vi "Lab Panel V5.24.2.vi"() -> ()   [LabVIEW 2013] (continued)
            n3236 = global read "Global display 3.vi" "log 1-1"() -> (→"LOG LAB01-1":string)
            n3237 = global read "Global display 3.vi" "log 3-1"() -> (→"LOG LAB03-1":string)
            n3238 = global read "Global display 3.vi" "log 1-2"() -> (→"LOG LAB01-2":string)
            n3239 = property on="Tab Control 2" class="TabCtl (strict)"() -> ("Pages"=w5991:refnum<vi>[])  [unwired: 2 in, 2 out]
            n3240 = global read "Global display 3.vi" "log 2-1"() -> (→"LOG LAB02-1":string)
            n3241 = global read "Global display 3.vi" "log 2-2"() -> (→"LOG LAB02-2":string)
            n3242 = global read "Global display 3.vi" "log 4-2"() -> (→"LOG LAB04-2":string)
            n3243 = global read "Global display 3.vi" "log 5-2"() -> (→"LOG LAB05-2":string)
            n3244 = global read "Global display 3.vi" "log 5-1"() -> (→"LOG LAB05-1":string)
            n3245 = global read "Global display 3.vi" "log 4-1"() -> (→"LOG LAB04-1":string)
            n3246 = global read "Global display 3.vi" "log 3-2"() -> (→"LOG LAB03-2":string)
            n3247 = Index Array(array=w5991, index=8) -> (element=w5989:refnum<vi>)
            n3248 = property class="Page"(reference=w5989) -> ("PageVis"=w5988:bool)  [unwired: 1 in, 2 out]
            n3249 = global write "Global display 3.vi" "admin"(w5988) -> ()
            n3250 = local read "O/I  LAB05-2"() -> (w6042:bool)
            n3251 = local read "O/I  LAB05-1"() -> (w6043:bool)
            n3252 = local read "O/I  LAB03-2"() -> (w6046:bool)
            n3253 = local read "O/I  LAB04-2"() -> (w6044:bool)
            n3254 = local read "O/I  LAB04-1"() -> (w6045:bool)
            n3255 = local read "O/I  LAB03-1"() -> (w6047:bool)
            n3256 = local read "O/I  LAB01-2"() -> (w6050:bool)
            n3257 = local read "O/I  LAB01-1"() -> (w6051:bool)
            n3258 = local read "O/I  LAB02-1"() -> (w6049:bool)
            n3259 = local read "O/I  LAB02-2"() -> (w6048:bool)
            n3260 = global write "Global display 1.vi" "5-2 O/F"(w6042) -> ()
            n3261 = global write "Global display 1.vi" "5-1 O/F"(w6043) -> ()
            n3262 = global write "Global display 1.vi" "4-1 O/F"(w6045) -> ()
            n3263 = global write "Global display 1.vi" "4-2 O/F"(w6044) -> ()
            n3264 = global write "Global display 1.vi" "3-2 O/F"(w6046) -> ()
            n3265 = global write "Global display 1.vi" "3-1 O/F"(w6047) -> ()
            n3266 = global write "Global display 1.vi" "2-2 O/F"(w6048) -> ()
            n3267 = global write "Global display 1.vi" "2-1 O/F"(w6049) -> ()
            n3268 = global write "Global display 1.vi" "1-2 O/F"(w6050) -> ()
            n3269 = global write "Global display 1.vi" "1-1 O/F"(w6051) -> ()
            n3270 = local read "TEMP START LAB02-2"() -> (w5974:cluster{"TL":dbl, "TN":dbl})
            n3271 = local read "run lab05-2"() -> (w6032:bool)
            n3272 = local read "TEMP START LAB01-2"() -> (w5976:cluster{"TL":dbl, "TN":dbl})
            n3273 = local read "TEMP START LAB02-1"() -> (w5975:cluster{"TL":dbl, "TN":dbl})
            n3274 = local read "TEMP START LAB04-1"() -> (w5971:cluster{"TL":dbl, "TN":dbl})
            n3275 = local read "TEMP START LAB04-2"() -> (w5970:cluster{"TL":dbl, "TN":dbl})
            n3276 = local read "run lab04-1"() -> (w6035:bool)
            n3277 = local read "run lab04-2"() -> (w6034:bool)
            n3278 = local read "run lab05-1"() -> (w6033:bool)
            n3279 = local read "TEMP START LAB01-1"() -> (w5977:cluster{"TL":dbl, "TN":dbl})
            n3280 = local read "TEMP START LAB05-2"() -> (w5968:cluster{"TL":dbl, "TN":dbl})
            n3281 = local read "TEMP START LAB05-1"() -> (w5969:cluster{"TL":dbl, "TN":dbl})
            n3282 = local read "run lab03-2"() -> (w6036:bool)
            n3283 = local read "TEMP START LAB03-2"() -> (w5972:cluster{"TL":dbl, "TN":dbl})
            n3284 = local read "TEMP START LAB03-1"() -> (w5973:cluster{"TL":dbl, "TN":dbl})
            n3285 = local read "run lab02-1"() -> (w6039:bool)
            n3286 = local read "run lab03-1"() -> (w6037:bool)
            n3287 = local read "run lab01-2"() -> (w6040:bool)
            n3288 = local read "run lab02-2"() -> (w6038:bool)
            n3289 = local read "run lab01-1"() -> (w6041:bool)
            n3290 = global write "Global display 1.vi" "5-2 R/S"(w6032) -> ()
            n3291 = global write "Global display 1.vi" "5-1 R/S"(w6033) -> ()
            n3292 = global write "Global display 1.vi" "4-2 R/S"(w6034) -> ()
            n3293 = global write "Global display 1.vi" "4-1 R/S"(w6035) -> ()
            n3294 = global write "Global display 1.vi" "3-2 R/S"(w6036) -> ()
            n3295 = global write "Global display 1.vi" "1-2 R/S"(w6040) -> ()
            n3296 = global write "Global display 1.vi" "2-1 R/S"(w6039) -> ()
            n3297 = global write "Global display 1.vi" "3-1 R/S"(w6037) -> ()
            n3298 = global write "Global display 1.vi" "2-2 R/S"(w6038) -> ()
            n3299 = global write "Global display 1.vi" "1-1 R/S"(w6041) -> ()
            n3300 = global write "Global display 3.vi" "TEMP ST 05-2"(w5968) -> ()
            n3301 = global write "Global display 3.vi" "TEMP ST 05-1"(w5969) -> ()
            n3302 = global write "Global display 3.vi" "TEMP ST 03-2"(w5972) -> ()
            n3303 = global write "Global display 3.vi" "TEMP ST 04-2"(w5970) -> ()
            n3304 = global write "Global display 3.vi" "TEMP ST 01-1"(w5977) -> ()
            n3305 = global write "Global display 3.vi" "TEMP ST 01-2"(w5976) -> ()
            n3306 = global write "Global display 3.vi" "TEMP ST 04-1"(w5971) -> ()
            n3307 = global write "Global display 3.vi" "TEMP ST 02-1"(w5975) -> ()
            n3308 = global write "Global display 3.vi" "TEMP ST 02-2"(w5974) -> ()
            n3309 = global write "Global display 3.vi" "TEMP ST 03-1"(w5973) -> ()
            n3310 = local read "DISP LAB04-2"() -> (w6024:T4)
            n3311 = local read "DISP LAB05-1"() -> (w6023:T4)
            n3312 = local read "DISP LAB04-1"() -> (w6025:T4)
            n3313 = local read "DISP LAB05-2"() -> (w6022:T4)
            n3314 = local read "DISP LAB03-1"() -> (w6027:T4)
            n3315 = local read "DISP LAB03-2"() -> (w6026:T4)
            n3316 = local read "DISP LAB01-2"() -> (w6030:T4)
            n3317 = local read "DISP LAB02-1"() -> (w6029:T4)
            n3318 = local read "DISP LAB02-2"() -> (w6028:T4)
            n3319 = local read "DISP LAB01-1"() -> (w6031:T4)
            n3320 = local read "TEMP RISE LAB05-1"() -> (w5959:cluster{"TL":dbl, "TN":dbl})
            n3321 = local read "TEMP RISE LAB05-2"() -> (w5958:cluster{"TL":dbl, "TN":dbl})
            n3322 = local read "TEMP RISE LAB04-2"() -> (w5960:cluster{"TL":dbl, "TN":dbl})
            n3323 = local read "TEMP RISE LAB04-1"() -> (w5961:cluster{"TL":dbl, "TN":dbl})
            n3324 = local read "TEMP RISE LAB03-2"() -> (w5962:cluster{"TL":dbl, "TN":dbl})
            n3325 = local read "TEMP RISE LAB03-1"() -> (w5963:cluster{"TL":dbl, "TN":dbl})
            n3326 = local read "TEMP RISE LAB01-2"() -> (w5966:cluster{"TL":dbl, "TN":dbl})
            n3327 = local read "TEMP RISE LAB02-2"() -> (w5964:cluster{"TL":dbl, "TN":dbl})
            n3328 = local read "TEMP RISE LAB01-1"() -> (w5967:cluster{"TL":dbl, "TN":dbl})
            n3329 = local read "TEMP RISE LAB02-1"() -> (w5965:cluster{"TL":dbl, "TN":dbl})
            n3330 = global write "Global display 2.vi" "DISP LAB05-1"(w6023) -> ()
            n3331 = global write "Global display 2.vi" "DISP LAB05-2"(w6022) -> ()
            n3332 = global write "Global display 2.vi" "DISP LAB04-2"(w6024) -> ()
            n3333 = global write "Global display 2.vi" "DISP LAB02-1"(w6029) -> ()
            n3334 = global write "Global display 2.vi" "DISP LAB02-2"(w6028) -> ()
            n3335 = global write "Global display 2.vi" "DISP LAB04-1"(w6025) -> ()
            n3336 = global write "Global display 2.vi" "DISP LAB01-2"(w6030) -> ()
            n3337 = global write "Global display 2.vi" "DISP LAB01-1"(w6031) -> ()
            n3338 = global write "Global display 2.vi" "DISP LAB03-1"(w6027) -> ()
            n3339 = global write "Global display 2.vi" "DISP LAB03-2"(w6026) -> ()
            n3340 = global write "Global display 3.vi" "TEMP RS 05-2"(w5958) -> ()
            n3341 = global write "Global display 3.vi" "TEMP RS 05-1"(w5959) -> ()
            n3342 = global write "Global display 3.vi" "TEMP RS 03-2"(w5962) -> ()
            n3343 = global write "Global display 3.vi" "TEMP RS 02-1"(w5965) -> ()
            n3344 = global write "Global display 3.vi" "TEMP RS 02-2"(w5964) -> ()
            n3345 = global write "Global display 3.vi" "TEMP RS 04-2"(w5960) -> ()
            n3346 = global write "Global display 3.vi" "TEMP RS 01-2"(w5966) -> ()
            n3347 = global write "Global display 3.vi" "TEMP RS 03-1"(w5963) -> ()
            n3348 = global write "Global display 3.vi" "TEMP RS 04-1"(w5961) -> ()
            n3349 = global write "Global display 3.vi" "TEMP RS 01-1"(w5967) -> ()
            n3350 = local read "SET LAB05-2"() -> (w6012:T5)
            n3351 = local read "SET LAB05-1"() -> (w6013:T5)
            n3352 = local read "SET LAB04-1"() -> (w6015:T5)
            n3353 = local read "SET LAB04-2"() -> (w6014:T5)
            n3354 = local read "SET LAB03-1"() -> (w6017:T5)
            n3355 = local read "SET LAB03-2"() -> (w6016:T5)
            n3356 = local read "SET LAB02-2"() -> (w6018:T5)
            n3357 = local read "SET LAB01-2"() -> (w6020:T5)
            n3358 = local read "SET LAB02-1"() -> (w6019:T5)
            n3359 = local read "SET LAB01-1"() -> (w6021:T5)
            n3360 = global write "Global display 2.vi" "SET LAB05-2"(w6012) -> ()
            n3361 = global write "Global display 2.vi" "SET LAB05-1"(w6013) -> ()
            n3362 = global write "Global display 2.vi" "SET LAB04-1"(w6015) -> ()
            n3363 = global write "Global display 2.vi" "SET LAB04-2"(w6014) -> ()
            n3364 = global write "Global display 2.vi" "SET LAB03-2"(w6016) -> ()
            n3365 = global write "Global display 2.vi" "SET LAB02-2"(w6018) -> ()
            n3366 = global write "Global display 2.vi" "SET LAB03-1"(w6017) -> ()
            n3367 = global write "Global display 2.vi" "SET LAB01-2"(w6020) -> ()
            n3368 = global write "Global display 2.vi" "SET LAB01-1"(w6021) -> ()
            n3369 = global write "Global display 2.vi" "SET LAB02-1"(w6019) -> ()
            n3370 = local read "RESULT LAB01-1"() -> (w6011:bool)
            n3371 = local read "RESULT LAB03-2"() -> (w6006:bool)
            n3372 = local read "RESULT LAB04-1"() -> (w6005:bool)
            n3373 = local read "RESULT LAB04-2"() -> (w6004:bool)
            n3374 = local read "RESULT LAB02-2"() -> (w6008:bool)
            n3375 = local read "RESULT LAB01-2"() -> (w6010:bool)
            n3376 = local read "RESULT LAB02-1"() -> (w6009:bool)
            n3377 = local read "RESULT LAB03-1"() -> (w6007:bool)
            n3378 = local read "RESULT LAB05-1"() -> (w6003:bool)
            n3379 = local read "RESULT LAB05-2"() -> (w6002:bool)
            n3380 = global write "Global display 2.vi" "RESULT LAB05-1"(w6003) -> ()
            n3381 = global write "Global display 2.vi" "RESULT LAB01-2"(w6010) -> ()
            n3382 = global write "Global display 2.vi" "RESULT LAB03-2"(w6006) -> ()
            n3383 = global write "Global display 2.vi" "RESULT LAB04-1"(w6005) -> ()
            n3384 = global write "Global display 2.vi" "RESULT LAB04-2"(w6004) -> ()
            n3385 = global write "Global display 2.vi" "RESULT LAB05-2"(w6002) -> ()
            n3386 = global write "Global display 2.vi" "RESULT LAB03-1"(w6007) -> ()
            n3387 = global write "Global display 2.vi" "RESULT LAB02-1"(w6009) -> ()
            n3388 = global write "Global display 2.vi" "RESULT LAB02-2"(w6008) -> ()
            n3389 = global write "Global display 2.vi" "RESULT LAB01-1"(w6011) -> ()
          }
          frame #22 {
            # "simulate values"
            n3390 = global write "Global display 4.vi" "LAB deg C"("LAB deg C") -> ()
          }
          frame #23 {
            # "end main and display program"
            n3391 = stacked-sequence {
              seq-local: [_ w6056 _] -> [_ _ w6059]
              tunnel: w6053 -> [w6054 _ _]
              frame #0 {
                n3392 = case shown="True" w6054 {
                  frame False {
                  }
                  frame True {
                    n3393 = One Button Dialog(message="Excessive number of USB \nresets done, re-start program.") -> ()  [unwired: 1 in, 1 out]
                  }
                }
              }
              frame #1 {
                # "check for reset error"
                n3394 = local read "Reset Error"() -> (w6056:bool)
                n3395 = case shown="True" w6056 {
                  frame False {
                  }
                  frame True {
                    n3396 = One Button Dialog(message="USB Reset ERROR, program will be stopped.\nClose program, close windows, switch panel off\nand re power panel. If error persists seek help.") -> ()  [unwired: 1 in, 1 out]
                  }
                }
              }
              frame #2 {
                # "end labview session"
                n3397 = Or(x=w6059, y="stop all") -> (x .or. y?=w6058:bool)
                n3398 = Quit LabVIEW(quit? (T)=w6058) -> ()
                n3399 = global write "Global display 1.vi" "stop disp"(w6058) -> ()
              }
            }
          }
        }
        n3400 = node-c288() -> ()  [unwired: 1 in, 1 out]
        "loops" <- w336
      }
      n3401 = node-c288(w309) -> ()  [unwired: 1 out]
    }
  }
